vi "Begin.vi"(8 "error in":errorcluster) -> (0 "error out":errorcluster)   [LabVIEW 2016]
doc: "Called before other user functions, this VI is expected to open initial I/O refnums, load in file data, and do all program initialization. Notice that the <B>error out</B> terminal is simply used for data flow. Wiring it to other structures or subVIs ensures that this VI runs first."
uses:
  <vilib>/Rock Robotics/SystemInterfaces/DIO/FPGA_DIOPWMChannel.ctl
  <vilib>/Rock Robotics/WPI/SafetyOutput/WPI_SafetyOutputConfigMenu.ctl
  <vilib>/Rock Robotics/WPI/DriverStation/WPI_DriverStationRobotMode2.ctl
  <vilib>/Rock Robotics/WPI/Joystick/WPI_JoystickDeviceEnum.ctl
  <vilib>/Rock Robotics/SystemInterfaces/DIO/FPGA_DIOChannel.ctl
  <vilib>/Rock Robotics/SystemInterfaces/AI/FPGA_AIGyroChannel.ctl
  <vilib>/Rock Robotics/WPI/Solenoid/WPI_SolenoidChannel.ctl
  <vilib>/Rock Robotics/WPI/RobotDrive/WPI_RobotDriveOpen2MotorWithSPARK.vi
  Robot Global Data.vi
  <vilib>/Rock Robotics/Network Tables/NT Write String Array.vi
  <vilib>/Rock Robotics/WPI/MotorControl/WPI_MotorControlOpen SPARK.vi
  <vilib>/Rock Robotics/WPI/Counter/WPI_CounterDigitalInputToDigitalSource.vi
  <vilib>/Rock Robotics/WPI/Gyro/WPI_GyroAnalogOpen.vi
  <vilib>/Rock Robotics/WPI/Solenoid/WPI_SolenoidOpenDouble.vi
  <vilib>/Rock Robotics/WPI/Utilities/WPI_GetSetVariantRefNum.vi
  <vilib>/Rock Robotics/WPI/Encoder/WPI_EncoderType.ctl
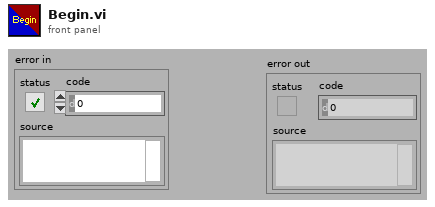
[diagram p1: front panel]
types:
  T1 = typedef "WPI_SolenoidChannel.ctl" = enum8{"Solenoid 0", "Solenoid 1", "Solenoid 2", "Solenoid 3", "Solenoid 4", "Solenoid 5", "Solenoid 6", "Solenoid 7", "Invalid"}
  T2 = typedef "FPGA_AIGyroChannel.ctl" = enum8{"AI 0", "AI 1", "Invalid"}
  T3 = typedef "WPI_JoystickDeviceEnum.ctl" = enum16{"USB 0", "USB 1", "USB 2", "USB 3", "USB 4", "USB 5"}
  T4 = typedef "FPGA_DIOChannel.ctl" = enum8{"DIO 0", "DIO 1", "DIO 2", "DIO 3", "DIO 4", "DIO 5", "DIO 6", "DIO 7", "DIO 8", "DIO 9", "DIO MXP 0", "DIO MXP 1", "DIO MXP 2", "DIO MXP 3", "DIO MXP 4", "DIO MXP 5", "DIO MXP 6", "DIO MXP 7", "DIO MXP 8", "DIO MXP 9", "DIO MXP 10", "DIO MXP 11", "DIO MXP 12", "DIO MXP 13", "DIO MXP 14", "DIO MXP 15", "SPI Port CS1", "SPI Port CS2", "SPI Port CS3", "SPI Port MISO", "SPI Port MOSI", "Invalid"}
  T5 = typedef "FPGA_DIOPWMChannel.ctl" = enum8{"PWM 0", "PWM 1", "PWM 2", "PWM 3", "PWM 4", "PWM 5", "PWM 6", "PWM 7", "PWM 8", "PWM 9", "PWM MXP 0", "PWM MXP 1", "PWM MXP 2", "PWM MXP 3", "PWM MXP 4", "PWM MXP 5", "PWM MXP 6", "PWM MXP 7", "PWM MXP 8", "PWM MXP 9", "Invalid"}
  T6 = typedef "WPI_DriverStationRobotMode2.ctl" = enum16{"Autonomous Disabled", "Autonomous Enabled", "Teleop Disabled", "Teleop Enabled", "Disconnected", "Finish", "Test Disabled", "Test Enabled", "Emergency Stopped"}
  T7 = typedef "WPI_SafetyOutputConfigMenu.ctl" = enum16{"Enable", "Disable"}
  T8 = typedef "WPI_DigitalInputDevRef.ctl" = cluster{"DevStatus":errorcluster, "DIO Channel":T4}
  T9 = typedef "FPGA_CounterEncoderSourceConvertionLVSourceType.ctl" = cluster{"DevStatus":errorcluster, "AnalogTriggerMode?":bool, "DigitalMode":cluster{"DIO Channel":T10}, "AnalogTriggerMode":cluster{"AnalogTriggerIndex":T11, "OutputType":T12}}
  T10 = typedef "FPGA_DIODigitalSourceChannel.ctl" = enum8{"DIO 0", "DIO 1", "DIO 2", "DIO 3", "DIO 4", "DIO 5", "DIO 6", "DIO 7", "DIO 8", "DIO 9", "DIO MXP 0", "DIO MXP 1", "DIO MXP 2", "DIO MXP 3", "DIO MXP 4", "DIO MXP 5", "DIO MXP 6", "DIO MXP 7", "DIO MXP 8", "DIO MXP 9", "DIO MXP 10", "DIO MXP 11", "DIO MXP 12", "DIO MXP 13", "DIO MXP 14", "DIO MXP 15", "Disabled"}
  T11 = typedef "FPGA_AnalogTriggerIndex.ctl" = enum8{"Trig 0", "Trig 1", "Trig 2", "Trig 3", "Trig 4", "Trig 5", "Trig 6", "Trig 7", "Invalid"}
  T12 = typedef "FPGA_AnalogTriggerOutType.ctl" = enum16{"InWindow", "TriggerState", "Rising", "Falling"}
  T13 = typedef "WPI_EncoderDevRef.ctl" = cluster{"DevStatus":errorcluster, "EncoderIndex":T14, "CounterIndex":T15, "DistancePerCount":dbl, "Decoding Type":T16}
  T14 = typedef "FPGA_EncoderIdx.ctl" = enum8{"Enc 0", "Enc 1", "Enc 2", "Enc 3", "Enc 4", "Enc 5", "Enc 6", "Enc 7", "Invalid"}
  T15 = typedef "FPGA_CounterCtrSystemIndex.ctl" = enum8{"Ctr 0", "Ctr 1", "Ctr 2", "Ctr 3", "Ctr 4", "Ctr 5", "Ctr 6", "Ctr 7", "Invalid"}
  T16 = typedef "WPI_EncoderType.ctl" = enum16{"1x", "2x", "4x"}
  T17 = typedef "WPI_CameraDevRef.ctl" = cluster{"Camera Address":string, "CameraStatus":errorcluster}
  T18 = typedef "WPI_GyroDevRef.ctl" = cluster{"DevStatus":errorcluster, "Analog Channel":T19, "Offset":dbl, "Gain (VoltsPerDegree/Second)":dbl, "Gyro Type":enum16{"Analog", "XRS450"}, "Handle":i32, "SPI Bus":T20, "Device Found":bool, "Sample Rate":dbl, "Calibrate On Open":bool}
  T19 = typedef "FPGA_AIChannel.ctl" = enum8{"AI 0", "AI 1", "AI 2", "AI 3", "AI MXP 0", "AI MXP 1", "AI MXP 2", "AI MXP 3", "Invalid"}
  T20 = typedef "spi_bus.ctl" = enum16{"SPI On-Board, CS0", "SPI On-Board, CS1", "SPI On-Board, CS2", "SPI On-Board, CS3", "SPI MXP", "Invalid"}
  T21 = typedef "WPI_JoystickDevRef.ctl" = cluster{"Device":T3}
  T22 = typedef "WPI_RobotDriveDevRef.ctl" = cluster{"DevStatus":errorcluster, "Motors[]":T23[], "Square Inputs":bool, "Max Output":dbl}
  T23 = typedef "WPI_MotorControlDeviceRef.ctl" = cluster{"DeviceStatus":errorcluster, "Type":T24, "PWM":cluster{"PWM Channel":T5, "DeadBand":T25}, "CAN":cluster{"Device Number":u8, "SetOutput VI Ref":variant, "GetOutput VI Ref":variant, "Enable VI Ref":variant, "Disable VI Ref":variant, "Data":variant}, "Invert":bool}
  T24 = typedef "WPI_MotorControlType.ctl" = enum16{"PWM", "CAN"}
  T25 = typedef "WPI_PWMDeadband.ctl" = cluster{"Name":string, "maxPositivePwm":i32, "minPositivePwm":i32, "centerPwm":i32, "maxNegativePwm":i32, "minNegativePwm":i32, "angularRange":u16}
  T26 = typedef "WPI_CompressorDevRef.ctl" = cluster{"DevStatus":errorcluster, "Pneumatics Control Module":u8}
  T27 = typedef "WPI_SolenoidDevRef.ctl" = cluster{"DevStatus":errorcluster, "Pneumatics Control Module":u8, "Forward Solenoid Channel":T1, "Reverse Solenoid Channel":T1}
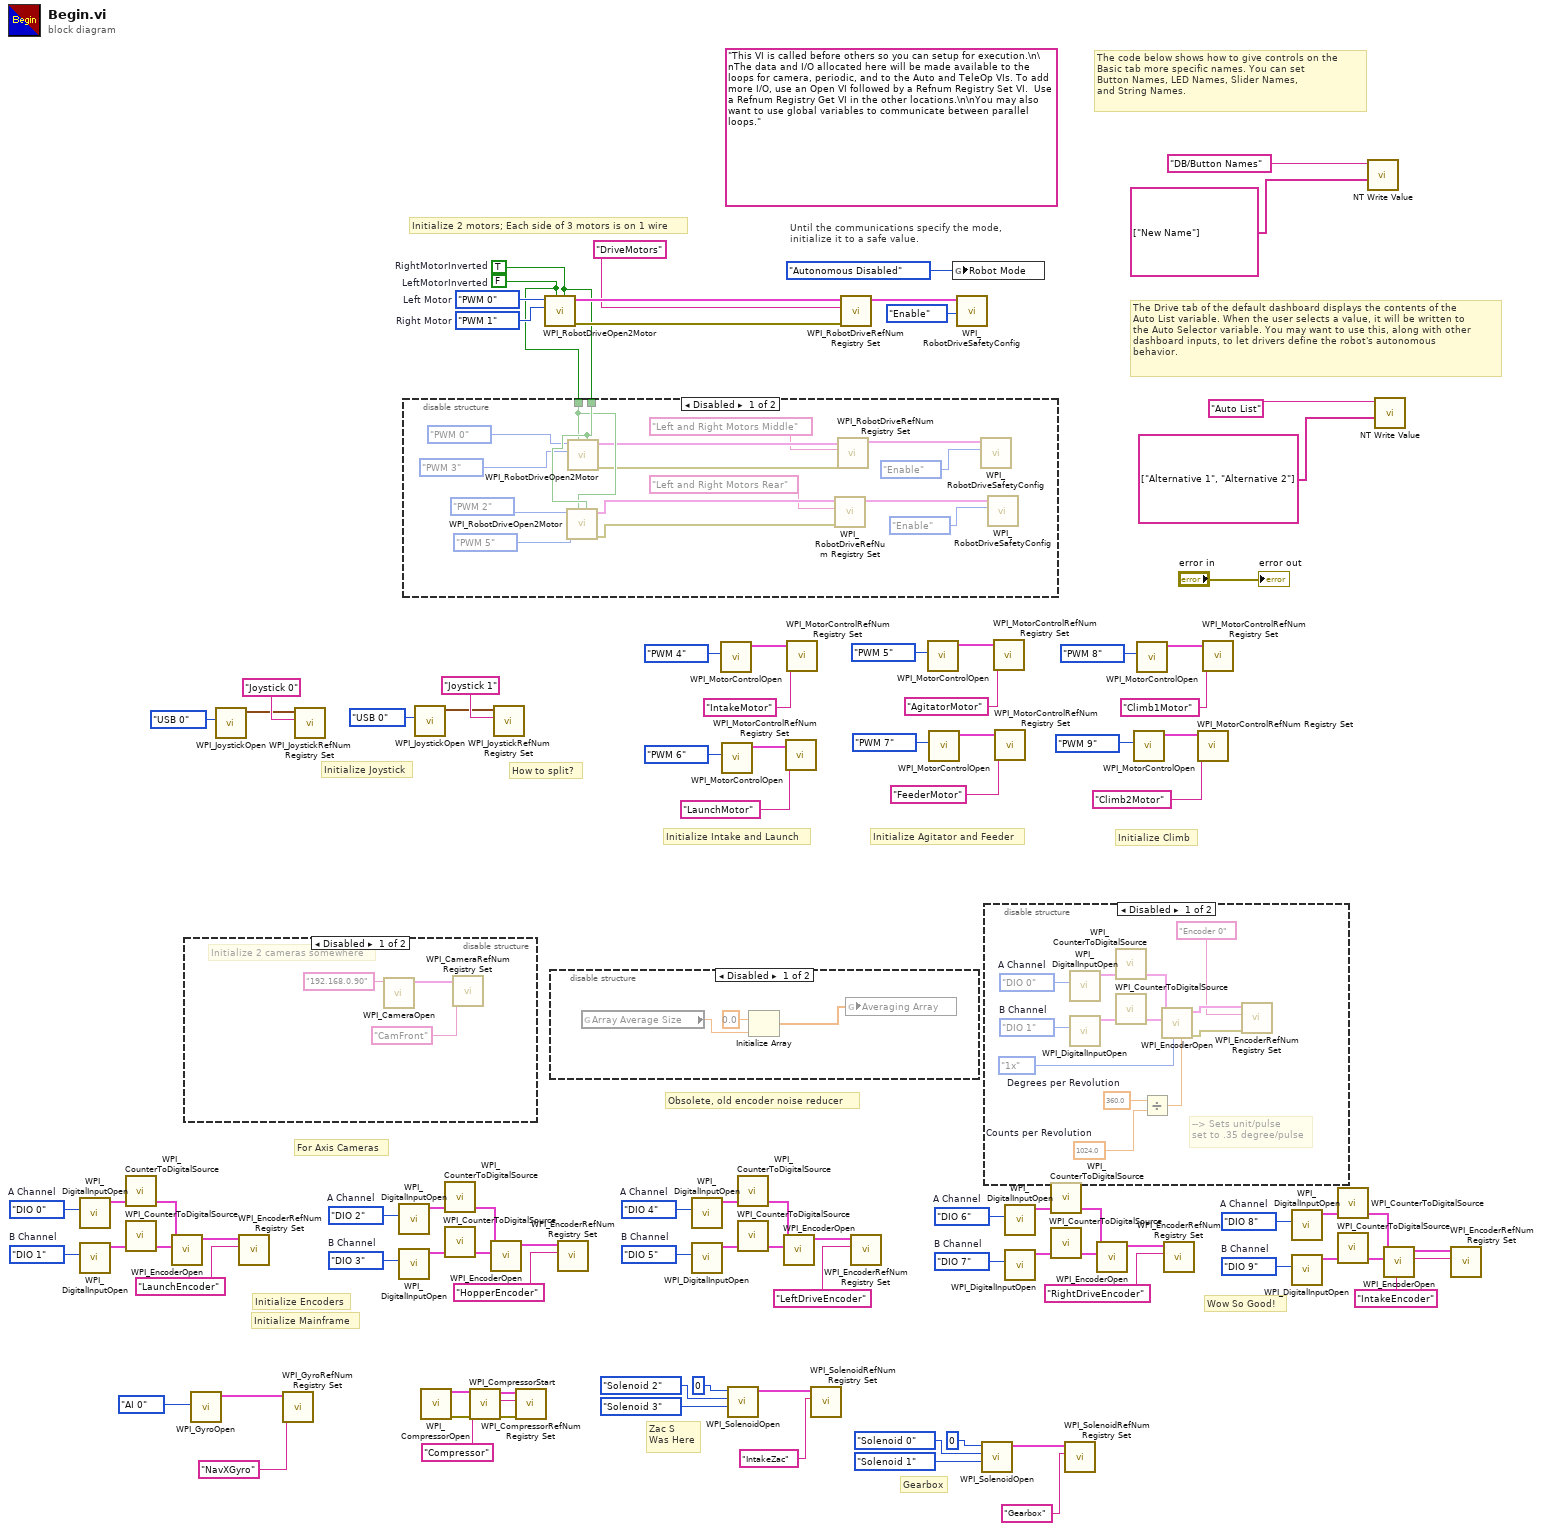
[diagram p0: block diagram]
diagram:
  w29 = FPGA_DIOChannel."DIO 9"  # B Channel
  w28 = FPGA_DIOChannel."DIO 8"  # A Channel
  w37 = FPGA_DIOChannel."DIO 7"  # B Channel
  w36 = FPGA_DIOChannel."DIO 6"  # A Channel
  w45 = FPGA_DIOChannel."DIO 5"  # B Channel
  w44 = FPGA_DIOChannel."DIO 4"  # A Channel
  w53 = FPGA_DIOChannel."DIO 3"  # B Channel
  w52 = FPGA_DIOChannel."DIO 2"  # A Channel
  w61 = FPGA_DIOChannel."DIO 1"  # B Channel
  w60 = FPGA_DIOChannel."DIO 0"  # A Channel
  (unwired) "This VI is called before others so you can setup for execution.\n\nThe data and I/O allocated here will be made available to the loops for camera, periodic, and to the Auto and TeleOp VIs. To add more I/O, use an Open VI followed by a Refnum Registry Set VI.  Use a Refnum Registry Get VI in the other locations.\n\nYou may also want to use global variables to communicate between parallel loops."
  w93 = FPGA_DIOPWMChannel."PWM 1"  # Right Motor
  w94 = FPGA_DIOPWMChannel."PWM 0"  # Left Motor
  w77 = FALSE  # LeftMotorInverted
  w78 = TRUE  # RightMotorInverted
  # "Gearbox"
  # "Initialize Mainframe"
  # "Wow So Good!"
  # "Zac S\nWas Here"
  # "How to split?"
  # "Initialize Encoders"
  # "Initialize Climb"
  # "Initialize Agitator and Feeder"
  # "For Axis Cameras"
  # "Obsolete, old encoder noise reducer"
  # "Initialize Intake and Launch"
  # "The Drive tab of the default dashboard displays the contents of the\nAuto List variable. When the user selects a value, it will be written to\nthe Auto Selector variable. You may want to use this, along with other\ndashboard inputs, to let drivers define the robot's autonomous\nbehavior."
  # "The code below shows how to give controls on the\nBasic tab more specific names. You can set\nButton Names, LED Names, Slider Names,\nand String Names."
  # "Initialize Joystick"
  # "Until the communications specify the mode,\ninitialize it to a safe value."
  # "Initialize 2 motors; Each side of 3 motors is on 1 wire"
  n1 = call <vilib>:"WPI_DigitalInputOpen.vi"("DIO Channel"=w60) -> ("DigitalInputDevRef"=w57:T8)  [unwired: 1 in, 9 out]
  n2 = call <vilib>:"WPI_DigitalInputOpen.vi"("DIO Channel"=w61) -> ("DigitalInputDevRef"=w58:T8)  [unwired: 1 in, 9 out]
  n3 = call-poly <vilib>:"WPI_CounterToDigitalSource.vi"("DigitalInputDevRef"=w57) -> ("Digital Source"=w56:T9)  [unwired: 6 out]
  n4 = call-poly <vilib>:"WPI_CounterToDigitalSource.vi"("DigitalInputDevRef"=w58) -> ("Digital Source"=w59:T9)  [unwired: 6 out]
  n5 = call <vilib>:"WPI_EncoderOpen.vi"("BSource"=w59, "ASource"=w56) -> ("EncoderDevRef"=w55:T13)  [unwired: 6 in, 3 out]
  n6 = disable-structure shown="Disabled" {
    frame Disabled {
      # "Initialize 2 cameras somewhere"
      n7 = call <vilib>:"WPI_CameraOpen.vi"("Camera Address"="192.168.0.90") -> ("CameraDevRef"=w100:T17)  [unwired: 9 in, 1 out]
      n8 = call <vilib>:"WPI_CameraRefNum Registry Set.vi"("refnum name"="CamFront", "CameraDevRef"=w100) -> ()  [unwired: 8 in, 2 out]
    }
    frame Enabled {
    }
  }
  n9 = call-poly <vilib>:"WPI_GyroOpen.vi"("Analog Channel"=FPGA_AIGyroChannel."AI 0") -> ("GyroDevRef"=w17:T18)  [unwired: 8 in, 2 out]
  n10 = call <vilib>:"WPI_JoystickOpen.vi"("JoystickDevice"=WPI_JoystickDeviceEnum."USB 0") -> ("JoystickDevRef"=w88:T21)  [unwired: 10 in]
  n11 = call <vilib>:"WPI_EncoderRefNum Registry Set.vi"("refnum name"="LaunchEncoder", "EncoderDevRef"=w55) -> ()  [unwired: 8 in, 2 out]
  n12 = call <vilib>:"WPI_GyroRefNum Registry Set.vi"("refnum name"="NavXGyro", "GyroDevRef"=w17) -> ()  [unwired: 8 in, 2 out]
  n13 = call <vilib>:"WPI_JoystickRefNum Registry Set.vi"("refnum name"="Joystick 0", "JoystickDevRef"=w88) -> ()  [unwired: 8 in, 2 out]
  n14 = call <vilib>:"WPI_DigitalInputOpen.vi"("DIO Channel"=w52) -> ("DigitalInputDevRef"=w49:T8)  [unwired: 1 in, 9 out]
  n15 = call <vilib>:"WPI_DigitalInputOpen.vi"("DIO Channel"=w53) -> ("DigitalInputDevRef"=w50:T8)  [unwired: 1 in, 9 out]
  n16 = disable-structure shown="Disabled" {
    disable-tunnel: w78 -> [w116 _]
    disable-tunnel: w77 -> [w115 _]
    frame Disabled {
      n17 = call-poly <vilib>:"WPI_RobotDriveOpen2Motor.vi"("Right Motor Inverted"=w116, "Left Motor Inverted"=w115, "Right Motor"=FPGA_DIOPWMChannel."PWM 5", "Left Motor"=FPGA_DIOPWMChannel."PWM 2") -> ("error out"=w108:errorcluster, "RobotDriveDevRef"=w110:T22)  [unwired: 1 in, 5 out]
      n18 = call-poly <vilib>:"WPI_RobotDriveOpen2Motor.vi"("Right Motor Inverted"=w116, "Left Motor Inverted"=w115, "Right Motor"=FPGA_DIOPWMChannel."PWM 3", "Left Motor"=FPGA_DIOPWMChannel."PWM 0") -> ("error out"=w107:errorcluster, "RobotDriveDevRef"=w109:T22)  [unwired: 1 in, 5 out]
      n19 = call <vilib>:"WPI_RobotDriveRefNum Registry Set.vi"("error in (no error)"=w108, "refnum name"="Left and Right Motors Rear", "RobotDriveDevRef"=w110) -> ("RobotDriveDevRef"=w111:T22)  [unwired: 1 in, 7 out]
      n20 = call <vilib>:"WPI_RobotDriveRefNum Registry Set.vi"("error in (no error)"=w107, "refnum name"="Left and Right Motors Middle", "RobotDriveDevRef"=w109) -> ("RobotDriveDevRef"=w112:T22)  [unwired: 1 in, 7 out]
      n21 = call <vilib>:"WPI_RobotDriveSafetyConfig.vi"("mode"=WPI_SafetyOutputConfigMenu."Enable", "RobotDriveDevRef"=w112) -> ()  [unwired: 8 in, 2 out]
      n22 = call <vilib>:"WPI_RobotDriveSafetyConfig.vi"("mode"=WPI_SafetyOutputConfigMenu."Enable", "RobotDriveDevRef"=w111) -> ()  [unwired: 8 in, 2 out]
    }
    frame Enabled {
    }
  }
  n23 = call <vilib>:"WPI_JoystickOpen.vi"("JoystickDevice"=WPI_JoystickDeviceEnum."USB 0") -> ("JoystickDevRef"=w20:T21)  [unwired: 10 in]
  n24 = call <vilib>:"WPI_CompressorOpen.vi"() -> ("CompressorDevRef"=w15:T26, "error out"=w13:errorcluster)  [unwired: 14 in]
  n25 = call-poly <vilib>:"WPI_CounterToDigitalSource.vi"("DigitalInputDevRef"=w49) -> ("Digital Source"=w48:T9)  [unwired: 6 out]
  n26 = call-poly <vilib>:"WPI_CounterToDigitalSource.vi"("DigitalInputDevRef"=w50) -> ("Digital Source"=w51:T9)  [unwired: 6 out]
  n27 = call <vilib>:"WPI_CompressorStart.vi"("error in (no error)"=w13, "CompressorDevRef"=w15) -> ("error out"=w12:errorcluster, "CompressorDevRef"=w14:T26)  [unwired: 8 in]
  n28 = call <vilib>:"WPI_EncoderOpen.vi"("BSource"=w51, "ASource"=w48) -> ("EncoderDevRef"=w47:T13)  [unwired: 6 in, 3 out]
  n29 = call <vilib>:"WPI_JoystickRefNum Registry Set.vi"("refnum name"="Joystick 1", "JoystickDevRef"=w20) -> ()  [unwired: 8 in, 2 out]
  n30 = call <vilib>:"WPI_CompressorRefNum Registry Set.vi"("error in (no error)"=w12, "refnum name"="Compressor", "CompressorDevRef"=w14) -> ()  [unwired: 7 in, 2 out]
  n31 = call-poly <vilib>:"WPI_RobotDriveOpen2Motor.vi"("Right Motor Inverted"=w78, "Left Motor Inverted"=w77, "Right Motor"=w93, "Left Motor"=w94) -> ("error out"=w95:errorcluster, "RobotDriveDevRef"=w97:T22)  [unwired: 1 in, 5 out]
  n32 = disable-structure shown="Disabled" {
    frame Disabled {
      n33 = global read "Robot Global Data.vi" "Array Average Size"() -> (w119:dbl)
      n34 = Initialize Array(0.0 ("element"), w119) -> (w117:dbl[])
      n35 = global write "Robot Global Data.vi" "Averaging Array"(w117) -> ()
    }
    frame Enabled {
    }
  }
  n36 = call <vilib>:"WPI_EncoderRefNum Registry Set.vi"("refnum name"="HopperEncoder", "EncoderDevRef"=w47) -> ()  [unwired: 8 in, 2 out]
  n37 = call <vilib>:"WPI_DigitalInputOpen.vi"("DIO Channel"=w44) -> ("DigitalInputDevRef"=w41:T8)  [unwired: 1 in, 9 out]
  n38 = call <vilib>:"WPI_DigitalInputOpen.vi"("DIO Channel"=w45) -> ("DigitalInputDevRef"=w42:T8)  [unwired: 1 in, 9 out]
  n39 = call-poly <vilib>:"WPI_MotorControlOpen.vi"("PWM Channel"=FPGA_DIOPWMChannel."PWM 4") -> ("MotorControlDeviceRef"=w75:T23)  [unwired: 9 in, 1 out]
  n40 = call-poly <vilib>:"WPI_MotorControlOpen.vi"("PWM Channel"=FPGA_DIOPWMChannel."PWM 6") -> ("MotorControlDeviceRef"=w80:T23)  [unwired: 9 in, 1 out]
  n41 = call-poly <vilib>:"WPI_SolenoidOpen.vi"("Reverse Solenoid Channel"=WPI_SolenoidChannel."Solenoid 3" ("Forward Solenoid Channel"), "Forward Solenoid Channel"=WPI_SolenoidChannel."Solenoid 2" ("Solenoid Channel"), "Pneumatics Control Module (0)"=u8 0) -> ("SolenoidDevRef"=w8:T27)  [unwired: 7 in, 1 out]
  n42 = call-poly <vilib>:"WPI_CounterToDigitalSource.vi"("DigitalInputDevRef"=w41) -> ("Digital Source"=w40:T9)  [unwired: 6 out]
  n43 = call-poly <vilib>:"WPI_CounterToDigitalSource.vi"("DigitalInputDevRef"=w42) -> ("Digital Source"=w43:T9)  [unwired: 6 out]
  n44 = call <vilib>:"WPI_EncoderOpen.vi"("BSource"=w43, "ASource"=w40) -> ("EncoderDevRef"=w39:T13)  [unwired: 6 in, 3 out]
  n45 = call <vilib>:"WPI_MotorControlRefNum Registry Set.vi"("refnum name"="LaunchMotor", "MotorControlDevRef"=w80) -> ()  [unwired: 8 in, 2 out]
  n46 = call <vilib>:"WPI_MotorControlRefNum Registry Set.vi"("refnum name"="IntakeMotor", "MotorControlDevRef"=w75) -> ()  [unwired: 8 in, 2 out]
  n47 = call <vilib>:"WPI_SolenoidRefNum Registry Set.vi"("refnum name"="IntakeZac", "SolenoidDevRef"=w8) -> ()  [unwired: 8 in, 2 out]
  n48 = call <vilib>:"WPI_RobotDriveRefNum Registry Set.vi"("error in (no error)"=w95, "refnum name"="DriveMotors", "RobotDriveDevRef"=w97) -> ("RobotDriveDevRef"=w92:T22)  [unwired: 1 in, 7 out]
  n49 = call <vilib>:"WPI_EncoderRefNum Registry Set.vi"("refnum name"="LeftDriveEncoder", "EncoderDevRef"=w39) -> ()  [unwired: 8 in, 2 out]
  n50 = call-poly <vilib>:"WPI_MotorControlOpen.vi"("PWM Channel"=FPGA_DIOPWMChannel."PWM 5") -> ("MotorControlDeviceRef"=w72:T23)  [unwired: 9 in, 1 out]
  n51 = call-poly <vilib>:"WPI_MotorControlOpen.vi"("PWM Channel"=FPGA_DIOPWMChannel."PWM 7") -> ("MotorControlDeviceRef"=w70:T23)  [unwired: 9 in, 1 out]
  n52 = global write "Robot Global Data.vi" "Robot Mode"(WPI_DriverStationRobotMode2."Autonomous Disabled" ("Robot Mode")) -> ()
  n53 = call <vilib>:"WPI_RobotDriveSafetyConfig.vi"("mode"=WPI_SafetyOutputConfigMenu."Enable", "RobotDriveDevRef"=w92) -> ()  [unwired: 8 in, 2 out]
  n54 = call-poly <vilib>:"WPI_SolenoidOpen.vi"("Reverse Solenoid Channel"=WPI_SolenoidChannel."Solenoid 1" ("Forward Solenoid Channel"), "Forward Solenoid Channel"=WPI_SolenoidChannel."Solenoid 0" ("Solenoid Channel"), "Pneumatics Control Module (0)"=u8 0) -> ("SolenoidDevRef"=w3:T27)  [unwired: 7 in, 1 out]
  n55 = disable-structure shown="Disabled" {
    frame Disabled {
      w120 = 360.0  # Degrees per Revolution
      w123 = 1024.0  # Counts per Revolution
      w132 = FPGA_DIOChannel."DIO 1"  # B Channel
      w131 = FPGA_DIOChannel."DIO 0"  # A Channel
      # "--> Sets unit/pulse\nset to .35 degree/pulse"
      n56 = call <vilib>:"WPI_DigitalInputOpen.vi"("DIO Channel"=w131) -> ("DigitalInputDevRef"=w128:T8)  [unwired: 1 in, 9 out]
      n57 = call <vilib>:"WPI_DigitalInputOpen.vi"("DIO Channel"=w132) -> ("DigitalInputDevRef"=w129:T8)  [unwired: 1 in, 9 out]
      n58 = call-poly <vilib>:"WPI_CounterToDigitalSource.vi"("DigitalInputDevRef"=w128) -> ("Digital Source"=w127:T9)  [unwired: 6 out]
      n59 = call-poly <vilib>:"WPI_CounterToDigitalSource.vi"("DigitalInputDevRef"=w129) -> ("Digital Source"=w130:T9)  [unwired: 6 out]
      n60 = Divide(x=w120, y=w123) -> (x/y=w122:dbl)
      n61 = call <vilib>:"WPI_EncoderOpen.vi"("DistancePerCount"=w122, "Decoding Type"=WPI_EncoderType."1x", "BSource"=w130, "ASource"=w127) -> ("error out"=w125:errorcluster, "EncoderDevRef"=w126:T13)  [unwired: 4 in, 2 out]
      n62 = call <vilib>:"WPI_EncoderRefNum Registry Set.vi"("error in (no error)"=w125, "refnum name"="Encoder 0", "EncoderDevRef"=w126) -> ()  [unwired: 7 in, 2 out]
    }
    frame Enabled {
    }
  }
  n63 = call <vilib>:"WPI_MotorControlRefNum Registry Set.vi"("refnum name"="AgitatorMotor", "MotorControlDevRef"=w72) -> ()  [unwired: 8 in, 2 out]
  n64 = call <vilib>:"WPI_MotorControlRefNum Registry Set.vi"("refnum name"="FeederMotor", "MotorControlDevRef"=w70) -> ()  [unwired: 8 in, 2 out]
  n65 = call <vilib>:"WPI_DigitalInputOpen.vi"("DIO Channel"=w36) -> ("DigitalInputDevRef"=w33:T8)  [unwired: 1 in, 9 out]
  n66 = call <vilib>:"WPI_DigitalInputOpen.vi"("DIO Channel"=w37) -> ("DigitalInputDevRef"=w34:T8)  [unwired: 1 in, 9 out]
  n67 = call-poly <vilib>:"WPI_CounterToDigitalSource.vi"("DigitalInputDevRef"=w33) -> ("Digital Source"=w32:T9)  [unwired: 6 out]
  n68 = call-poly <vilib>:"WPI_CounterToDigitalSource.vi"("DigitalInputDevRef"=w34) -> ("Digital Source"=w35:T9)  [unwired: 6 out]
  n69 = call <vilib>:"WPI_SolenoidRefNum Registry Set.vi"("refnum name"="Gearbox", "SolenoidDevRef"=w3) -> ()  [unwired: 8 in, 2 out]
  n70 = call <vilib>:"WPI_EncoderOpen.vi"("BSource"=w35, "ASource"=w32) -> ("EncoderDevRef"=w31:T13)  [unwired: 6 in, 3 out]
  n71 = call-poly <vilib>:"WPI_MotorControlOpen.vi"("PWM Channel"=FPGA_DIOPWMChannel."PWM 9") -> ("MotorControlDeviceRef"=w66:T23)  [unwired: 9 in, 1 out]
  n72 = call-poly <vilib>:"WPI_MotorControlOpen.vi"("PWM Channel"=FPGA_DIOPWMChannel."PWM 8") -> ("MotorControlDeviceRef"=w64:T23)  [unwired: 9 in, 1 out]
  n73 = call <vilib>:"WPI_EncoderRefNum Registry Set.vi"("refnum name"="RightDriveEncoder", "EncoderDevRef"=w31) -> ()  [unwired: 8 in, 2 out]
  n74 = call <vilib>:"WPI_MotorControlRefNum Registry Set.vi"("refnum name"="Climb2Motor", "MotorControlDevRef"=w66) -> ()  [unwired: 8 in, 2 out]
  n75 = call <vilib>:"WPI_MotorControlRefNum Registry Set.vi"("refnum name"="Climb1Motor", "MotorControlDevRef"=w64) -> ()  [unwired: 8 in, 2 out]
  n76 = call <vilib>:"WPI_DigitalInputOpen.vi"("DIO Channel"=w28) -> ("DigitalInputDevRef"=w25:T8)  [unwired: 1 in, 9 out]
  n77 = call <vilib>:"WPI_DigitalInputOpen.vi"("DIO Channel"=w29) -> ("DigitalInputDevRef"=w26:T8)  [unwired: 1 in, 9 out]
  n78 = call-poly <vilib>:"WPI_CounterToDigitalSource.vi"("DigitalInputDevRef"=w25) -> ("Digital Source"=w24:T9)  [unwired: 6 out]
  n79 = call-poly <vilib>:"WPI_CounterToDigitalSource.vi"("DigitalInputDevRef"=w26) -> ("Digital Source"=w27:T9)  [unwired: 6 out]
  n80 = call-poly <vilib>:"NT Write Value.vi"("String Array"=string[] ["New Name"], "Name"="DB/Button Names") -> ()  [unwired: 9 in, 1 out]
  n81 = call-poly <vilib>:"NT Write Value.vi"("String Array"=string[] ["Alternative 1", "Alternative 2"], "Name"="Auto List") -> ()  [unwired: 9 in, 1 out]
  n82 = call <vilib>:"WPI_EncoderOpen.vi"("BSource"=w27, "ASource"=w24) -> ("EncoderDevRef"=w23:T13)  [unwired: 6 in, 3 out]
  n83 = call <vilib>:"WPI_EncoderRefNum Registry Set.vi"("refnum name"="IntakeEncoder", "EncoderDevRef"=w23) -> ()  [unwired: 8 in, 2 out]
  "error out" <- "error in"
